vi "PH_IEEE1394Camera.configure Cam.vi"(0 "VI in":refnum<vi>, 2 "IMAQ1394 Session In":T1, 4 "Cam Error in":errorcluster, 5 "error in (no error)":errorcluster) -> (14 "VI out":refnum<vi>, 16 "IMAQ1394 Session Out":T1, 18 "Cam Error out":errorcluster, 19 "error out":errorcluster)   [LabVIEW 2014, in "PH_IEEE1394Camera.lvlib"]
uses:
  PH_IEEE1394Camera.lvlib
  <vilib>/userdefined/High Color/IMAQdx.ctl
  <vilib>/vision/driver/NI_Vision_Acquisition_Software.lvlib
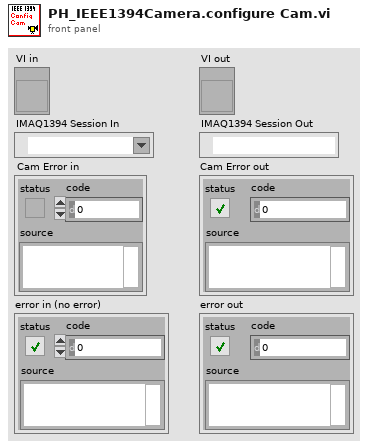
[diagram p1: front panel]
types:
  T1 = typedef "IMAQdx.ctl" = refnum<k21>
  T2 = cluster{"Name":string, "Num Value":dbl, "String Value":string, "Boolean Value":bool}[]
  T3 = typedef "PH_IEEE1394Camera.lvlib/PH_IEEE1394Camera.i attribute.ctl" = cluster{"Gui Refs":cluster{"Brightness":refnum<vi>, "Shutter":refnum<vi>, "Gain":refnum<vi>, "Center of Gravity":refnum<vi>, "Supported Video Modes":refnum<vi>, "Trigger Polarity":refnum<vi>, "Trigger Mode":refnum<vi>, "Trigger Timeout":refnum<vi>, "Bit Depth":refnum<vi>, "Video Mode":refnum<vi>, "Top":refnum<vi>, "Bottom":refnum<vi>, "Left":refnum<vi>, "Right":refnum<vi>, "Set ROI to Maximum":refnum<vi>, "Camera Details":refnum<vi>, "Current Cam Attributes":refnum<vi>, "Attribute to set":refnum<vi>, "Num Value":refnum<vi>, "String Value":refnum<vi>, "Bool Value":refnum<vi>, "Set Cam Attribute":refnum<vi>}, "Cam":cluster{"IMAQ1394 Session":T1, "Camera Details":T4}, "Current Attributes":T5[], "Supported Video Modes ":cluster{"Video Mode":u32, "Video Mode Name":string}[], "Wanted Attributes":cluster{"Name":string, "Num Value":dbl, "String Value":string, "Boolean Value":bool}[], "Cam Attributes":T7}
  T4 = typedef "PH_IEEE1394Camera.lvlib/PH_IEEE1394Camera.Cam Details.ctl" = cluster{"Model":string, "Serial Number":dbl, "Cam name (Machinery)":string, "Bus Type":string}
  T5 = typedef "PH_IEEE1394Camera.lvlib/PH_IEEE1394Camera.Cam Attribute.ctl" = cluster{"Information":cluster{"Type":T6, "Readable":bool, "Writable":bool, "Name":string}, "Num Value":dbl, "String Value":string, "Maximum":dbl, "Minimum":dbl, "Units":string, "Description":string, "EnumStrings[]":string[], "EnumValues[]":u32[], "Boolean Value":bool}
  T6 = typedef "NI_Vision_Acquisition_Software.lvlib/IMAQdx Attribute Type.ctl" = enum32{"U32", "I64", "DBL", "String", "Enum", "Bool", "Command"}
  T7 = typedef "PH_IEEE1394Camera.lvlib/PH_IEEE1394Camera.Relevant Cam Attributes.ctl" = cluster{"Video Mode":cluster{"Name":string, "Index":i32}, "Brightness":cluster{"Name":string, "Index":i32}, "Gain":cluster{"Name":string, "Index":i32}, "Shutter":cluster{"Name":string, "Index":i32}, "Trigger Pol":cluster{"Name":string, "Index":i32}, "Trigger Mode":cluster{"Name":string, "Index":i32}, "Timeout":cluster{"Name":string, "Index":i32}, "Bit Depth":cluster{"Name":string, "Index":i32}, "Pixel Bits":cluster{"Name":string, "Index":i32}, "Pixel Bytes":cluster{"Name":string, "Index":i32}, "Left":cluster{"Name":string, "Index":i32}, "Right":cluster{"Name":string, "Index":i32}, "Top":cluster{"Name":string, "Index":i32}, "Bottom":cluster{"Name":string, "Index":i32}}
  T8 = cluster{"Attribute Type":T6, "Readable":bool, "Writable":bool, "Attribute Name":string}[]
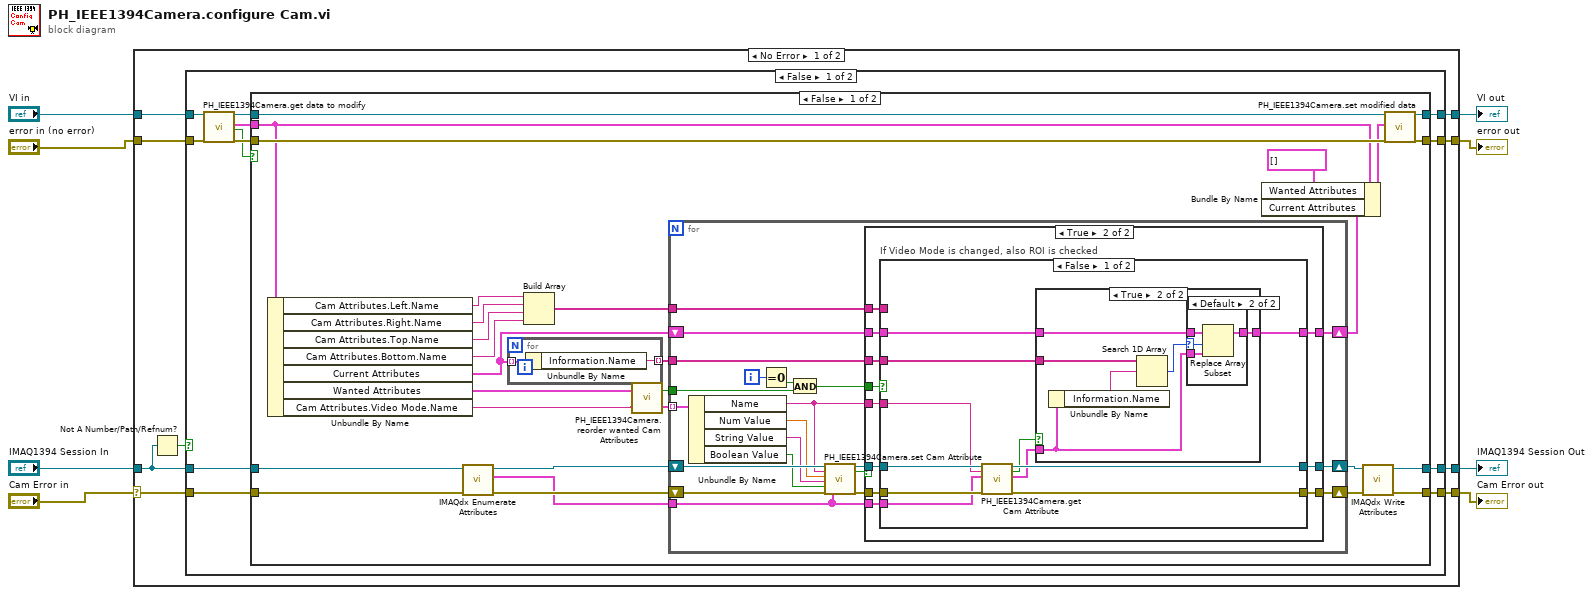
[diagram p0: block diagram]
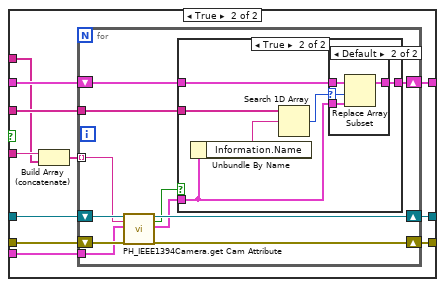
[diagram p5: hidden frame]
diagram:
  n1 = case shown="No Error" "Cam Error in" {
    selector: "Cam Error in" -> [w11 w160]
    tunnel: "IMAQ1394 Session In" -> [w10 w161]
    tunnel: "VI in" -> [w17 w163]
    tunnel: [w16 w161] -> w6
    tunnel: [w15 w163] -> w5
    tunnel: "error in (no error)" -> [w14 w162]
    tunnel: [w13 w162] -> w3
    tunnel: [w12 w160] -> w2
    frame No Error {
      n2 = Not A Number/Path/Refnum?(number/path/refnum=w10) -> (NaN/Path/Refnum?=w9:bool)
      n3 = case shown="False" w9 {
        tunnel: w10 -> [w29 w157]
        tunnel: w17 -> [w28 w159]
        tunnel: [w27 w157] -> w16
        tunnel: [w26 w159] -> w15
        tunnel: w14 -> [w25 w158]
        tunnel: [w24 w158] -> w13
        tunnel: [w23 w156] -> w12
        tunnel: w11 -> [w18 w156]
        frame False {
          n4 = call "PH_IEEE1394Camera.get data to modify.vi"("i ref in"=w28, "error in (no error)"=w25) -> ("i ref out"=w22:refnum<vi>, "i attribute"=w20:T3, "timed out"=w19:bool, "error out"=w21:errorcluster)  [unwired: 14 in]
          n5 = case shown="False" w19 {
            tunnel: w29 -> [w57 w153]
            tunnel: [w39 w153] -> w27
            tunnel: [w36 w155] -> w26
            tunnel: [w37 w154] -> w24
            tunnel: [w38 w152] -> w23
            tunnel: w18 -> [w56 w152]
            tunnel: w22 -> [w55 w155]
            tunnel: w21 -> [w54 w154]
            tunnel: w20 -> [w46 _]
            frame False {
              n6 = Unbundle By Name(w46) -> ("Cam Attributes.Left.Name"=w42:string, "Cam Attributes.Right.Name"=w41:string, "Cam Attributes.Top.Name"=w40:string, "Cam Attributes.Bottom.Name"=w35:string, "Current Attributes"=w31:T5[], "Wanted Attributes"=w32:T2, "Cam Attributes.Video Mode.Name"=w30:string)
              n7 = call <vilib>:"IMAQdx Enumerate Attributes.vi"("error in"=w56, "Session In"=w57) -> ("error out"=w52:errorcluster, "Attribute Information Array"=w49:T8, "Session Out"=w53:T1)  [unwired: 7 in]
              n8 = for {
                tunnel: w31 -> [w59] mode=indexing
                tunnel: [w58] -> w34 mode=indexing
                n9 = Unbundle By Name(w59) -> ("Information.Name"=w58:string)
              }
              n10 = Build Array(w42, w41, w40, w35) -> (w33:string[])
              n11 = call "PH_IEEE1394Camera.reorder wanted Cam Attributes.vi"("Name of Cam Attribute \"Video Mode\""=w30, "Wanted Attributes"=w32) -> ("redordered Wanted Attributes"=w44:T2, "Video Mode is going to be changed and at first array position"=w43:bool)
              n12 = for {
                tunnel: w49 -> [w73]
                shift-right: [w77] -> w51
                shift-left: w53 -> [w80]
                shift-right: [w75] -> w50
                shift-left: w52 -> [w79]
                shift-right: [w72] -> w45
                shift-left: w31 -> [w67]
                tunnel: w44 -> [w71] mode=indexing
                tunnel: w43 -> [w62]
                tunnel: w33 -> [w65]
                tunnel: w34 -> [w60]
                i -> [w64]
                n13 = Unbundle By Name(w71) -> ("Name"=w66:string, "Num Value"=w70:dbl, "String Value"=w69:string, "Boolean Value"=w68:bool)
                n14 = Equal To 0?(x=w64) -> (x = 0?=w63:bool)
                n15 = And(x=w63, y=w62) -> (x .and. y?=w61:bool)
                n16 = call "PH_IEEE1394Camera.set Cam Attribute.vi"("IMAQ1394 Session In"=w80, "Cam Attribute Name"=w66, "Attribute Value Num"=w70, "Attribute String / Command"=w69, "Attribute Bool"=w68, "Cam Error in"=w79, "Attribute Information Array"=w73) -> ("IMAQ1394 Session Out"=w78:T1, "Attribute changed?"=w74:bool, "Cam Error out"=w76:errorcluster)  [unwired: 10 in]
                n17 = case shown="True" w74 {
                  tunnel: w78 -> [w82 w94]
                  tunnel: [w82 w93] -> w77
                  tunnel: w76 -> [w81 w92]
                  tunnel: [w81 w91] -> w75
                  tunnel: w73 -> [_ w90]
                  tunnel: [w83 w89] -> w72
                  tunnel: w67 -> [w83 w88]
                  tunnel: w60 -> [_ w87]
                  tunnel: w66 -> [_ w86]
                  tunnel: w61 -> [_ w85]
                  tunnel: w65 -> [_ w84]
                  frame False {
                  }
                  frame True {
                    n18 = case "If Video Mode is changed, also ROI is checked" shown="False" w85 {
                      tunnel: w94 -> [w105 w128]
                      tunnel: [w104 w127] -> w93
                      tunnel: w92 -> [w103 w126]
                      tunnel: [w102 w125] -> w91
                      tunnel: w90 -> [w101 w124]
                      tunnel: [w99 w123] -> w89
                      tunnel: w88 -> [w98 w122]
                      tunnel: w87 -> [w96 w119]
                      tunnel: w86 -> [w95 w121]
                      tunnel: w84 -> [_ w118]
                      frame False {
                        n19 = call "PH_IEEE1394Camera.get Cam Attribute.vi"("IMAQ1394 Session In"=w105, "Cam Attribute Name"=w95, "Attribute Information Array"=w101, "Cam Error in"=w103) -> ("IMAQ1394 Session Out"=w104:T1, "Attribute read?"=w97:bool, "Cam Attribute Value"=w100:T5, "Cam Error out"=w102:errorcluster)  [unwired: 12 in]
                        n20 = case shown="True" w97 {
                          tunnel: w100 -> [_ w110]
                          tunnel: [w106 w111] -> w99
                          tunnel: w98 -> [w106 w112]
                          tunnel: w96 -> [_ w109]
                          frame False {
                          }
                          frame True {
                            n21 = Unbundle By Name(w110) -> ("Information.Name"=w108:string)
                            n22 = Search 1D Array(1D array=w109, element=w108) -> (index of element=w107:i32)  [unwired: 1 in]
                            n23 = case shown="Default" w107 {
                              selector: w107 -> [_ w114]
                              tunnel: w112 -> [w113 w117]
                              tunnel: [w113 w116] -> w111
                              tunnel: w110 -> [_ w115]
                              frame -1 {
                              }
                              frame Default {
                                n24 = Replace Array Subset(array=w117, new element=w115, index=w114) -> (w116:T5[])
                              }
                            }
                          }
                        }
                      }
                      frame True {
                        n25 = Build Array (concatenate)(w121, w118) -> (w120:string[])
                        n26 = for {
                          tunnel: w124 -> [w135]
                          tunnel: w119 -> [w130]
                          tunnel: w120 -> [w129] mode=indexing
                          shift-right: [w138] -> w127
                          shift-left: w128 -> [w139]
                          shift-right: [w136] -> w125
                          shift-left: w126 -> [w137]
                          shift-right: [w133] -> w123
                          shift-left: w122 -> [w132]
                          n27 = call "PH_IEEE1394Camera.get Cam Attribute.vi"("IMAQ1394 Session In"=w139, "Cam Attribute Name"=w129, "Attribute Information Array"=w135, "Cam Error in"=w137) -> ("IMAQ1394 Session Out"=w138:T1, "Attribute read?"=w131:bool, "Cam Attribute Value"=w134:T5, "Cam Error out"=w136:errorcluster)  [unwired: 12 in]
                          n28 = case shown="True" w131 {
                            tunnel: w134 -> [_ w144]
                            tunnel: [w140 w145] -> w133
                            tunnel: w132 -> [w140 w146]
                            tunnel: w130 -> [_ w143]
                            frame False {
                            }
                            frame True {
                              n29 = Unbundle By Name(w144) -> ("Information.Name"=w142:string)
                              n30 = Search 1D Array(1D array=w143, element=w142) -> (index of element=w141:i32)  [unwired: 1 in]
                              n31 = case shown="Default" w141 {
                                selector: w141 -> [_ w148]
                                tunnel: w146 -> [w147 w151]
                                tunnel: [w147 w150] -> w145
                                tunnel: w144 -> [_ w149]
                                frame -1 {
                                }
                                frame Default {
                                n32 = Replace Array Subset(array=w151, new element=w149, index=w148) -> (w150:T5[])
                                }
                              }
                            }
                          }
                        }
                      }
                    }
                  }
                }
              }
              n33 = Bundle By Name(cluster=w46, "Wanted Attributes"=T2 [], "Current Attributes"=w45) -> (w48:T3)
              n34 = call <vilib>:"IMAQdx Write Attributes.vi"("error in"=w50, "Session In"=w51) -> ("error out"=w38:errorcluster, "Session Out"=w39:T1)  [unwired: 8 in]
              n35 = call "PH_IEEE1394Camera.set modified data.vi"("i ref in"=w55, "i attribute"=w48, "error in (no error)"=w54) -> ("i ref out"=w36:refnum<vi>, "error out"=w37:errorcluster)  [unwired: 15 in]
            }
            frame True {
            }
          }
        }
        frame True {
        }
      }
    }
    frame Error {
    }
  }
  "error out" <- w3
  "VI out" <- w5
  "IMAQ1394 Session Out" <- w6
  "Cam Error out" <- w2
